vi "Data_Write_Signal_To_Disk.vi"(7 "wfm info":T1, 8 "error in (no error)":errorcluster, 9 "filename":string, 10 "path":path, 11 "data":i16[](array[numeric])) -> (0 "error out":errorcluster)   [LabVIEW 2020]
doc: "This VI writes a raw dataset to a disk file with the following format :\n- number of points = one value (I16)\n- data = number of points values (I16)\n- 1/sample rate, i.e. time step = one value (DBL)\n- vertical range = one value (DBL)\n- offset = one value (DBL)\nCalibrated data are obtained with : data * vertical range + offset\n\nThe file naming convention is :\nyyyy_mm_dd_xxx.A00 for the first acqusisition,\nyyyy_mm_dd_xxx.B00 for the second, etc."
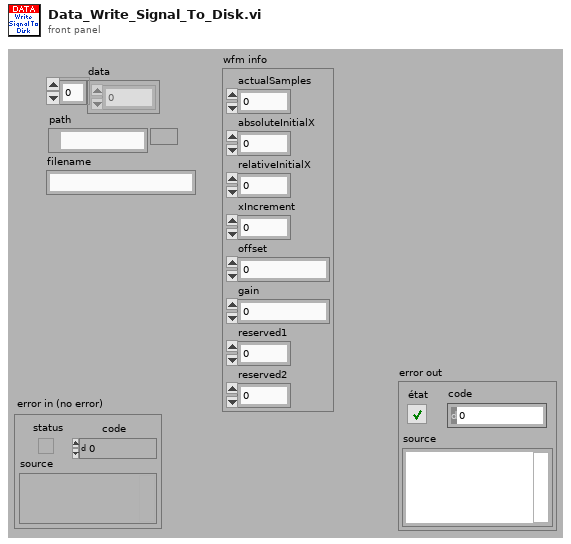
[diagram p1: front panel]
types:
  T1 = cluster{"actualSamples":i32, "absoluteInitialX":dbl, "relativeInitialX":dbl, "xIncrement":dbl, "offset":dbl, "gain":dbl, "reserved1":dbl, "reserved2":dbl}
  T2 = enum16{"big-endian, network order", "native, host order", "little-endian"}
  T3 = enum16{"open", "replace", "create", "open or create", "replace or create", "replace or create with confirmation"}
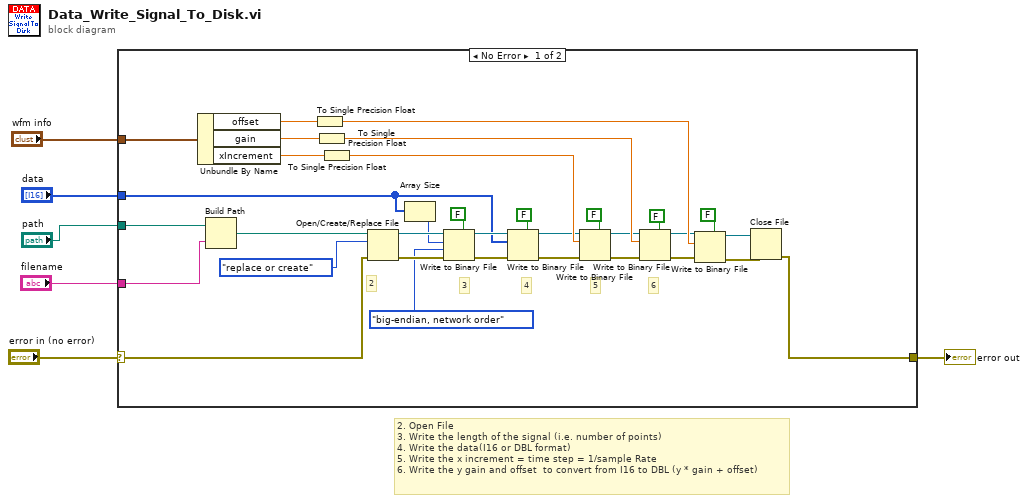
[diagram p0: block diagram]
diagram:
  # "2. Open File\n3. Write the length of the signal (i.e. number of points)\n4. Write the data(I16 or DBL format)\n5. Write the x increment = time step = 1/sample Rate\n6. Write the y gain and offset  to convert from I16 to DBL (y * gain + offset)"
  n1 = case shown="No Error" "error in (no error)" {
    selector: "error in (no error)" -> [w8 w40]
    tunnel: [w32 w40] -> w4
    tunnel: "wfm info" -> [w39 _]
    tunnel: "data" -> [w7 _]
    tunnel: "path" -> [w10 _]
    tunnel: "filename" -> [w9 _]
    frame No Error {
      # "2"
      # "6"
      # "5"
      # "4"
      # "3"
      n2 = Unbundle By Name(w39) -> ("offset"=w38:dbl, "gain"=w37:dbl, "xIncrement"=w36:dbl)
      n3 = Build Path(base path=w10, name or relative path=w9) -> (appended path=w29:path)
      n4 = To Single Precision Float(number=w38) -> (single precision float=w33:sgl)
      n5 = To Single Precision Float(number=w37) -> (single precision float=w34:sgl)
      n6 = To Single Precision Float(number=w36) -> (single precision float=w35:sgl)
      n7 = Open/Create/Replace File(file path (use dialog)=w29, error in=w8, operation (0:open)=T3."replace or create" ("opération (0 : open)")) -> (refnum out=w28:refnum<file>, error out=w27:errorcluster)  [unwired: 3 in, 1 out]
      n8 = Array Size(array=w7) -> (size(s)=w12:i32)
      n9 = Write to Binary File(file (use dialog)=w28, data=w12, error in=w27, 5:FALSE ("ajouter une taille de tableau ou de chaîne ? (V)"), 9:T2."big-endian, network order" ("ordre des octets (0 : big-Endian, network order)")) -> (refnum out=w24:refnum<file>, error out=w25:errorcluster)  [unwired: 1 in, 1 out]
      n10 = Write to Binary File(file (use dialog)=w24, data=w7, error in=w25, 5:FALSE ("ajouter une taille de tableau ou de chaîne ? (V)")) -> (refnum out=w22:refnum<file>, error out=w23:errorcluster)  [unwired: 2 in, 1 out]
      n11 = Write to Binary File(file (use dialog)=w22, data=w35, error in=w23, 5:FALSE ("ajouter une taille de tableau ou de chaîne ? (V)")) -> (refnum out=w19:refnum<file>, error out=w20:errorcluster)  [unwired: 2 in, 1 out]
      n12 = Write to Binary File(file (use dialog)=w19, data=w34, error in=w20, 5:FALSE ("ajouter une taille de tableau ou de chaîne ? (V)")) -> (refnum out=w16:refnum<file>, error out=w17:errorcluster)  [unwired: 2 in, 1 out]
      n13 = Write to Binary File(file (use dialog)=w16, data=w33, error in=w17, 5:FALSE ("ajouter une taille de tableau ou de chaîne ? (V)")) -> (refnum out=w15:refnum<file>, error out=w14:errorcluster)  [unwired: 2 in, 1 out]
      n14 = Close File(refnum=w15, error in=w14) -> (error out=w32:errorcluster)  [unwired: 1 out]
    }
    frame Error {
    }
  }
  "error out" <- w4
